vi "BLE_Notify_Listener.vi"(0 ".NET Refnum in":refnum<k24>, 5 "UUID":string, 7 "WriteByteArray":u8[](array[numeric]), 11 "error in (no error)":errorcluster) -> (4 ".NET Refnum out":refnum<k24>, 10 "Result":string, 15 "error out":errorcluster)   [LabVIEW 2019]
uses:
  C:/Users/chrismadlax/Desktop/LabVIEW-BLE-Driver/BLELib.dll
  BLELib.dll
panel:
  out "Numeric":i32
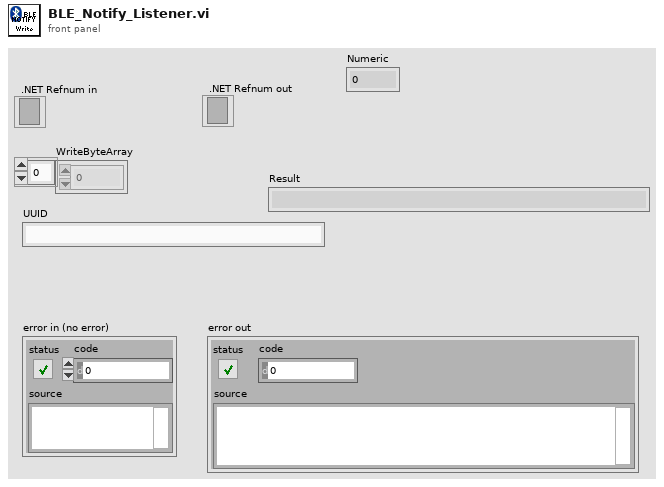
[diagram p1: front panel]
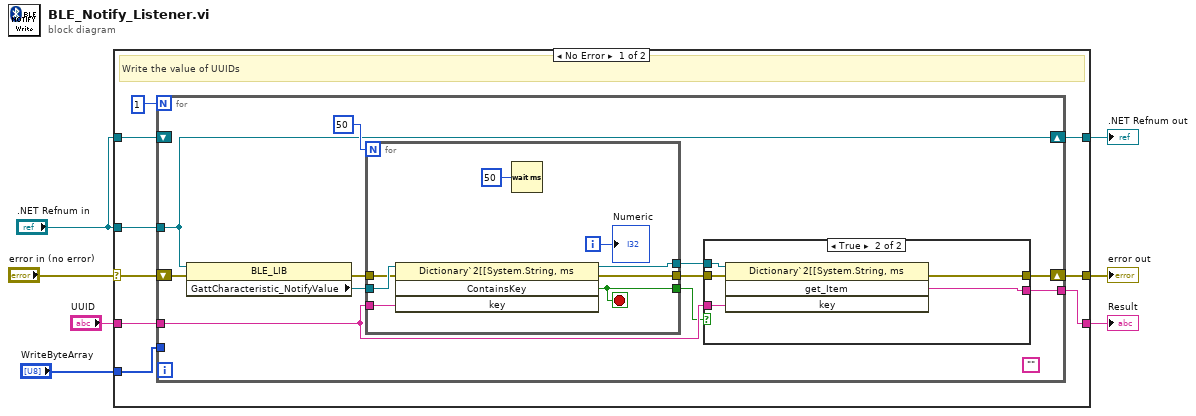
[diagram p0: block diagram]
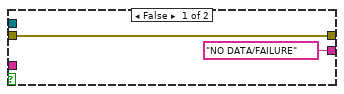
[diagram p2: hidden frame]
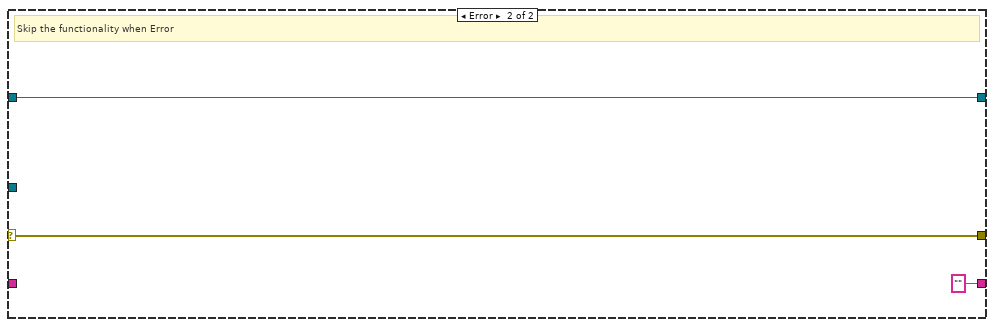
[diagram p3: hidden frame]
diagram:
  n1 = case shown="No Error" "error in (no error)" {
    selector: "error in (no error)" -> [w15 w45]
    tunnel: "UUID" -> [w9 _]
    tunnel: "WriteByteArray" -> [w16 _]
    tunnel: [w8 "" ("Result")] -> w5
    tunnel: [w14 w45] -> w3
    tunnel: [w13 w44] -> w2
    tunnel: ".NET Refnum in" -> [w12 w44]
    tunnel: ".NET Refnum in" -> [w10 _]
    frame No Error {
      # "Write the value of UUIDs"
      n2 = for {
        N: 1 -> [_]
        tunnel: w16 -> [_]
        shift-right: [w22] -> w14
        shift-left: w15 -> [w25]
        shift-right: [w18] -> w13
        shift-left: w12 -> [_]
        tunnel: w10 -> [w18]
        tunnel: w9 -> [w21]
        tunnel: [w20] -> w8
        (unwired) ""
        n3 = property class="BLE_LIB"(reference=w18, error in=w25) -> (error out=w24:errorcluster, "GattCharacteristic_NotifyValue"=w26:refnum<k24>)  [unwired: 1 out]
        n4 = for {
          N: 50 -> [_]
          tunnel: w26 -> [w42]
          tunnel: w21 -> [w41]
          tunnel: w24 -> [w40]
          tunnel: [w39] -> w23
          tunnel: [w38] -> w19
          tunnel: [w36] -> w17
          i -> [w37]
          stop <- w36 stop-if-true
          n5 = invoke class="Dictionary`2[[System.String, ms" method="ContainsKey"(reference=w42, error in=w40, "key"=w41) -> (reference out=w38:refnum<k24>, error out=w39:errorcluster, "ContainsKey"=w36:bool)  [unwired: 1 in, 1 out]
          n6 = Wait (ms)(milliseconds to wait=u32 50) -> ()  [unwired: 1 out]
          "Numeric" <- w37
        }
        n7 = case shown="True" w17 {
          tunnel: w23 -> [w28 w34]
          tunnel: [w28 w33] -> w22
          tunnel: w21 -> [_ w32]
          tunnel: ["NO DATA/FAILURE" ("get_Item") w31] -> w20
          tunnel: w19 -> [_ w30]
          frame False {
          }
          frame True {
            n8 = invoke class="Dictionary`2[[System.String, ms" method="get_Item"(reference=w30, error in=w34, "key"=w32) -> (error out=w33:errorcluster, "get_Item"=w31:string)  [unwired: 1 in, 2 out]
          }
        }
      }
    }
    frame Error {
      # "Skip the functionality when Error"
    }
  }
  "Result" <- w5
  "error out" <- w3
  ".NET Refnum out" <- w2
